vi "Write.vi"(0 "video writer in":refnum<class "MSC Video Writer.lvclass">, 1 "image in":refnum<class "MSC Image.lvclass">, 5 "error in (no error)":errorcluster) -> (14 "video writer out":refnum<class "MSC Video Writer.lvclass">, 15 "image out":refnum<class "MSC Image.lvclass">, 19 "error out":errorcluster)   [LabVIEW 2014, in "MSC Video Writer.lvclass"]
doc: "Writes a frame to the opened Video Writer object."
uses:
  MSC Video Writer.lvclass
  MSC Image_class/MSC Image.lvclass
  MSC Video Writer.lvclass/MSC Video Writer.ctl
  Dependencies/x86/MSC I Process32.dll
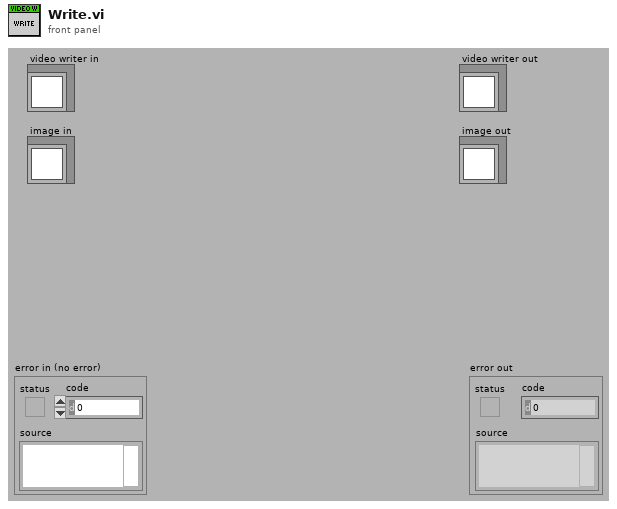
[diagram p1: front panel]
types:
  T1 = typedef "MSC Image.lvclass/Image.ctl" = cluster{"Pointer":u64, "Size":T2, "Image Type":T3, "Time Stamp":timestamp, "Variant":variant}
  T2 = typedef "MSC Image.lvclass/Size.ctl" = cluster{"Cols":i32, "Rows":i32}
  T3 = typedef "MSC Image.lvclass/Image Type.ctl" = i32
  T4 = typedef "MSC Video Writer.lvclass/Video Writer.ctl" = cluster{"Pointer":u64, "FPS":u32, "Path":path, "FourCC Codec":string, "Size":T2, "Type":T3}
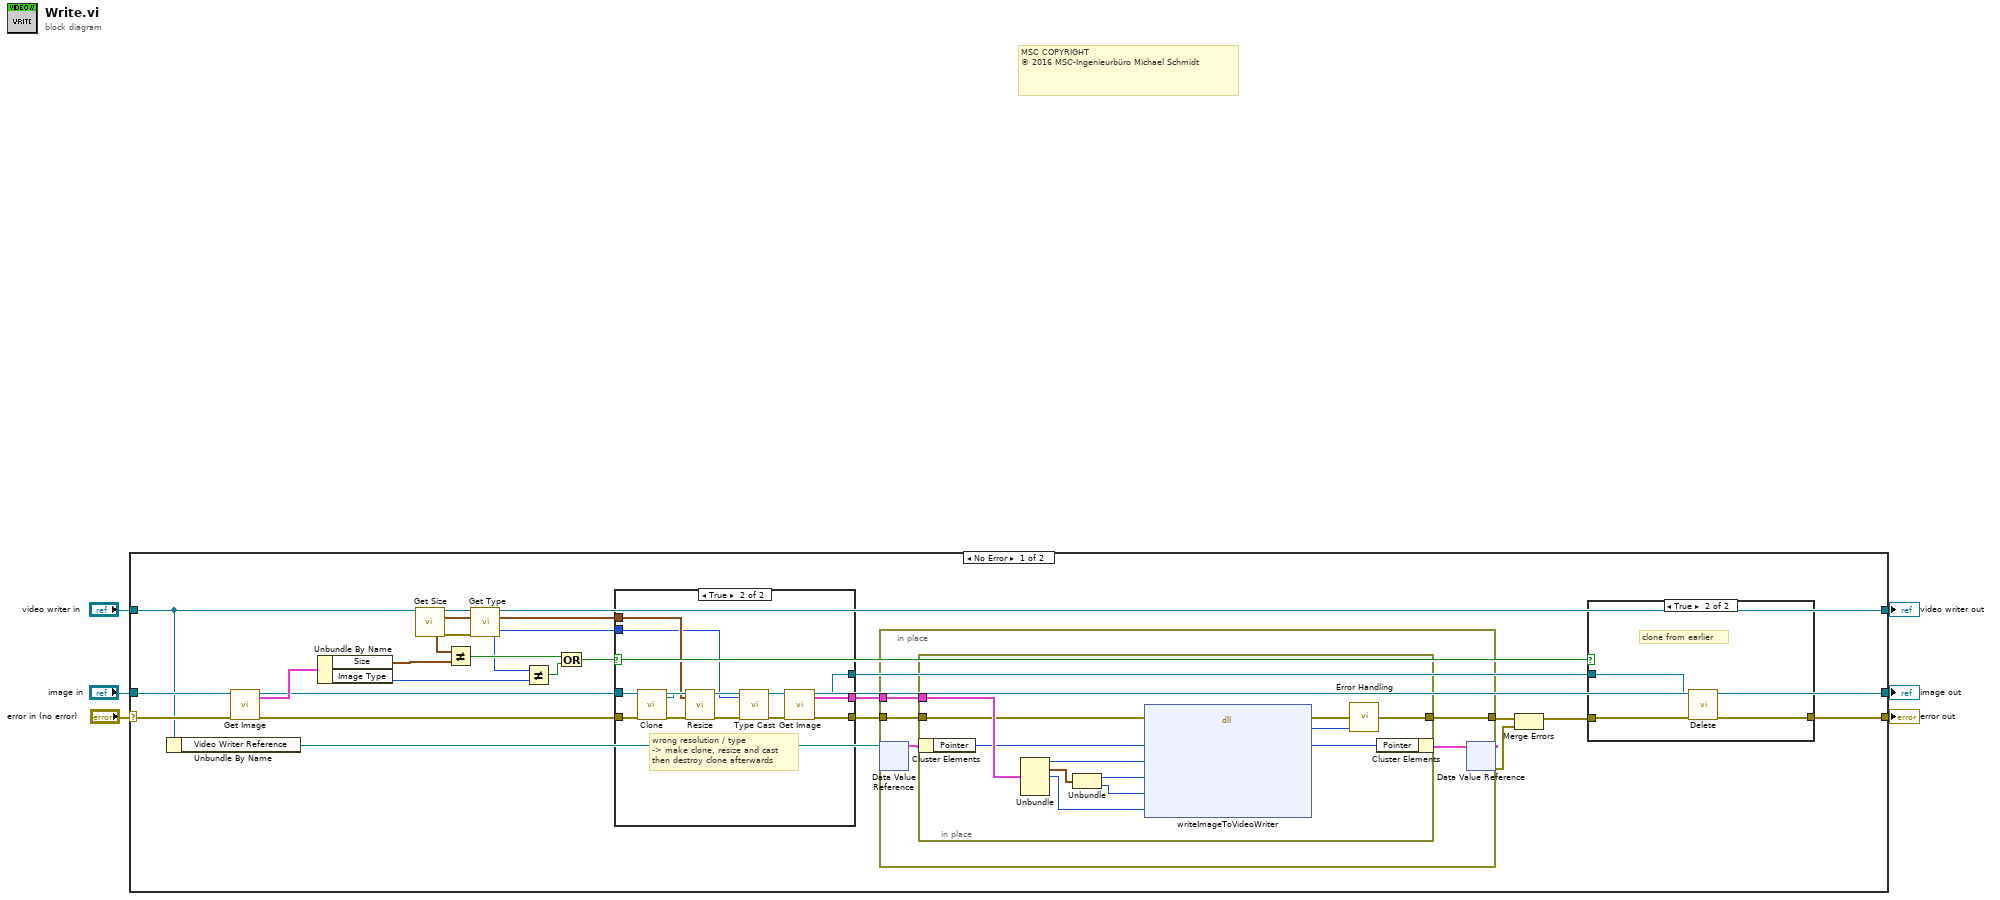
[diagram p0: block diagram]
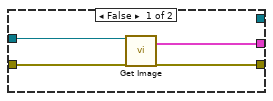
[diagram p3: hidden frame]
diagram:
  # "MSC COPYRIGHT\n© 2016 MSC-Ingenieurbüro Michael Schmidt"
  # "MSC COPYRIGHT\n© 2016 MSC-Ingenieurbüro Michael Schmidt"
  n1 = case shown="No Error" "error in (no error)" {
    selector: "error in (no error)" -> [w28 w71]
    tunnel: [w11 w71] -> w5
    tunnel: [w18 w70] -> w3
    tunnel: "video writer in" -> [w19 w70]
    tunnel: "image in" -> [w29 w69]
    tunnel: [w21 w69] -> w1
    frame No Error {
      n2 = Unbundle By Name(w19) -> ("Video Writer Reference"=w30:refnum<data-value>)
      n3 = call-dynamic "Get Image.vi"("image in"=w29, "error in (no error)"=w28) -> ("image out"=w21:refnum<class "MSC Image.lvclass">, "Image"=w26:T1, "error out"=w20:errorcluster)  [unwired: 15 in]
      n4 = Unbundle By Name(w26) -> ("Size"=w24:T2, "Image Type"=w25:T3)
      n5 = call-dynamic "Get Size.vi"("video writer in"=w19) -> ("video writer out"=w17:refnum<class "MSC Video Writer.lvclass">, "Size"=w14:T2, "error out"=w27:errorcluster)  [unwired: 16 in]
      n6 = Not Equal?(x=w14, y=w24) -> (x != y?=w23:bool)
      n7 = call-dynamic "Get Type.vi"("video writer in"=w17, "error in (no error)"=w27) -> ("video writer out"=w18:refnum<class "MSC Video Writer.lvclass">, "Type"=w13:T3)  [unwired: 15 in, 1 out]
      n8 = Not Equal?(x=w13, y=w25) -> (x != y?=w22:bool)
      n9 = Or(x=w23, y=w22) -> (x .or. y?=w7:bool)
      n10 = case shown="True" w7 {
        tunnel: w21 -> [w55 w68]
        tunnel: w20 -> [w54 w67]
        tunnel: [_ w57] -> w8
        tunnel: w14 -> [_ w64]
        tunnel: w13 -> [_ w63]
        tunnel: [w52 w58] -> w10
        tunnel: [w53 w56] -> w9
        frame False {
          n11 = call-dynamic "Get Image.vi"("image in"=w55, "error in (no error)"=w54) -> ("Image"=w52:T1, "error out"=w53:errorcluster)  [unwired: 15 in, 1 out]
        }
        frame True {
          # "wrong resolution / type\n-> make clone, resize and cast\nthen destroy clone afterwards"
          n12 = call-dynamic "Clone.vi"("image in"=w68, "error in (no error)"=w67) -> ("clone image out"=w65:refnum<class "MSC Image.lvclass">, "error out"=w62:errorcluster)  [unwired: 15 in, 1 out]
          n13 = call-dynamic "Resize.vi"("image in"=w65, "Size"=w64, "error in (no error)"=w62) -> ("image out"=w66:refnum<class "MSC Image.lvclass">, "error out"=w61:errorcluster)  [unwired: 15 in]
          n14 = call-dynamic "Type Cast.vi"("image in"=w66, "Image Type"=w63, "error in (no error)"=w61) -> ("image out"=w60:refnum<class "MSC Image.lvclass">, "error out"=w59:errorcluster)  [unwired: 15 in]
          n15 = call-dynamic "Get Image.vi"("image in"=w60, "error in (no error)"=w59) -> ("image out"=w57:refnum<class "MSC Image.lvclass">, "Image"=w58:T1, "error out"=w56:errorcluster)  [unwired: 15 in]
        }
      }
      n16 = in-place {
        in-place-border: [w37] -> w15
        in-place-border: w9 -> [w36]
        in-place-border: w10 -> [w35]
        n17 = in-place-dvr #1(w30) -> (w38:T4)  [unwired: 1 out]
        n18 = in-place {
          in-place-border: [w46] -> w37
          in-place-border: w36 -> [w49]
          in-place-border: w35 -> [w51]
          n19 = in-place-cluster #2(w38) -> ("Pointer"=w41:u64)
          n20 = Unbundle(w51) -> ("Pointer"=w45:u64, "Size"=w50:T2, "Image Type"=w42:T3)  [unwired: 2 out]
          n21 = Unbundle(w50) -> ("Cols"=w44:i32, "Rows"=w43:i32)
          n22 = dll-call lib="C:/Users/MSC/LabVIEW Projekte/LV 2014/MSC I-Process/user.lib/MSC-I Process/Dependencies/x86/MSC I Process*.dll" fn="writeImageToVideoWriter"(error in=w49, "writerPointer"=w41, "pointer"=w45, "cols"=w44, "rows"=w43, "type"=w42) -> (error out=w47:errorcluster, "error"=w48:i32, "writerPointer"=w40:u64)  [unwired: 6 in, 1 out]
          n23 = call "Error Handling.vi"("error in (no error)"=w47, "return type"=w48) -> ("error out"=w46:errorcluster)  [unwired: 12 in, 1 out]
          n24 = in-place-cluster #2("Pointer"=w40) -> (w39:T4)
        }
        n25 = in-place-dvr #1(w39) -> (w16:errorcluster)  [unwired: 1 out]
      }
      n26 = Merge Errors(w15, w16) -> (w12:errorcluster)
      n27 = case shown="True" w7 {
        tunnel: w12 -> [w31 w34]
        tunnel: [w31 w33] -> w11
        tunnel: w8 -> [_ w32]
        frame False {
        }
        frame True {
          # "clone from earlier"
          n28 = call-dynamic "Delete.vi"("image in"=w32, "error in (no error)"=w34) -> ("error out"=w33:errorcluster)  [unwired: 17 in]
        }
      }
    }
    frame Error {
    }
  }
  "error out" <- w5
  "video writer out" <- w3
  "image out" <- w1
